vi "Get State Constant States.vi"(8 "error in (no error)":errorcluster, 11 "StrCnst Refnum":refnum<vi>) -> (0 "error out":errorcluster, 2 "States":string[](array[string]))   [LabVIEW 2020, in "JKI State Machine API.lvlib"]
uses:
  JKI State Machine API.lvlib
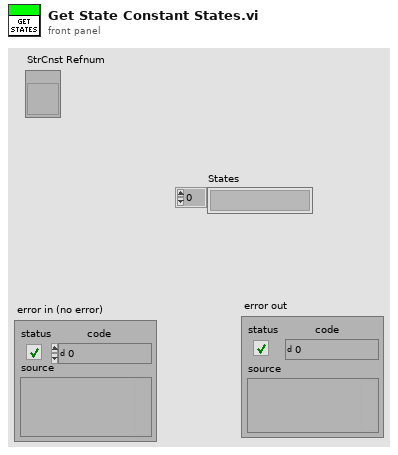
[diagram p1: front panel]
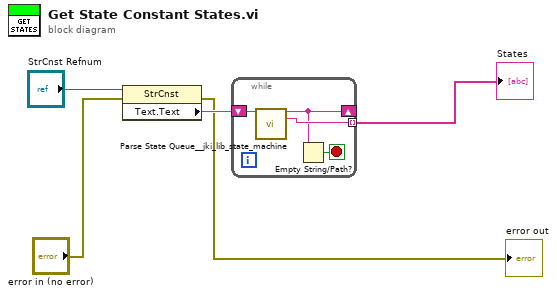
[diagram p0: block diagram]
diagram:
  n1 = property class="StrCnst"(reference="StrCnst Refnum", error in="error in (no error)") -> (error out=→"error out":errorcluster, "Text.Text"=w3:string)  [unwired: 1 out]
  n2 = while {
    shift-right: [w6] -> _
    shift-left: w3 -> [w9]
    tunnel: [w8] -> w1 mode=indexing
    stop <- w7 stop-if-true
    n3 = call <vilib>:"Parse State Queue__jki_lib_state_machine.vi"("State Queue"=w9) -> ("Remaining States"=w6:string, "Current State"=w8:string)  [unwired: 12 in, 1 out]
    n4 = Empty String/Path?(string/path=w6) -> (empty?=w7:bool)
  }
  "States" <- w1
